vi "Clear.vi"(8 "error in (no error)":errorcluster, 11 "CollectionByRef in":refnum<class "CollectionByRef.lvclass">) -> (0 "error out":errorcluster, 3 "CollectionByRef out":refnum<class "CollectionByRef.lvclass">)   [LabVIEW 2021, in "Collection.lvlib" / "CollectionByRef.lvclass"]
uses:
  CollectionByRef.lvclass
  CollectionByRef.lvclass/CollectionByRef.ctl
  CollectionByValue/CollectionByValue.lvclass
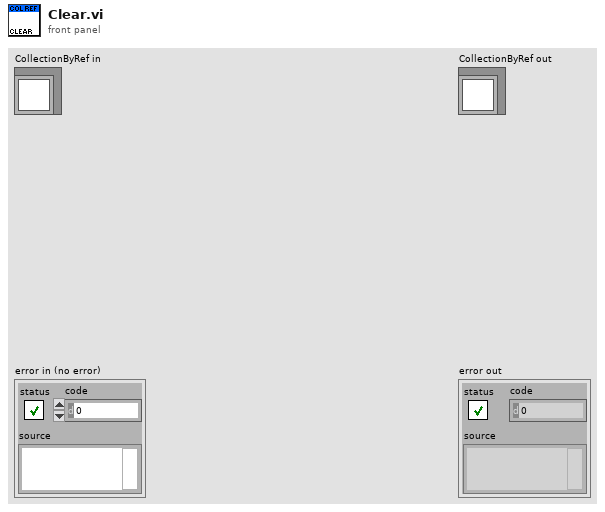
[diagram p1: front panel]
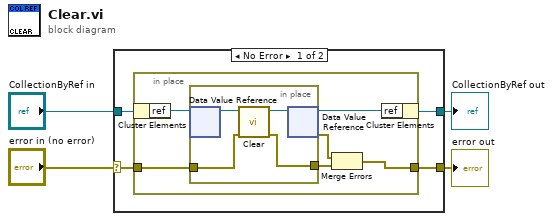
[diagram p0: block diagram]
diagram:
  n1 = case shown="No Error" "error in (no error)" {
    selector: "error in (no error)" -> [w6 w20]
    tunnel: [w5 w20] -> w1
    tunnel: [w7 w19] -> w3
    tunnel: "CollectionByRef in" -> [w8 w19]
    frame No Error {
      n2 = in-place {
        in-place-border: w6 -> [w12]
        in-place-border: [w9] -> w5
        n3 = in-place-cluster #1(w8) -> ("ref"=w13:refnum<data-value>)
        n4 = in-place {
          in-place-border: w12 -> [w16]
          in-place-border: [w15] -> w10
          n5 = in-place-dvr #2(w13) -> (w18:refnum<class "CollectionByValue.lvclass">)  [unwired: 1 out]
          n6 = call "Clear.vi"("error in (no error)"=w16, "Collection in"=w18) -> ("error out"=w15:errorcluster, "Collection out"=w17:refnum<class "CollectionByValue.lvclass">)  [unwired: 8 in]
          n7 = in-place-dvr #2(w17) -> (w14:refnum<data-value>, w11:errorcluster)
        }
        n8 = Merge Errors(w11, w10) -> (w9:errorcluster)
        n9 = in-place-cluster #1("ref"=w14) -> (w7:refnum<class "CollectionByRef.lvclass">)
      }
    }
    frame Error {
    }
  }
  "error out" <- w1
  "CollectionByRef out" <- w3
